vi "Read Temperature Controller Parameters.vi"(8 "error in (no error)":errorcluster, 11 "Temperature Controller Parameters in":refnum<class "Temperature Controller Parameters.lvclass">) -> (0 "error out":errorcluster, 2 "Data":T1={"Record heater"=FALSE, "Record RAW"=FALSE, "Set point"=0.0, "Heater range"=0.0, "Approach"=enum."Instant", "Ramp rate, K/min"=1.0, "Record Channels"=[], "Settling time "=60.0, "Settling range"=0.1, "P"=0.0, "I"=0.0, "D"=0.0, "Temperature Control"=FALSE}, 3 "Temperature Controller Parameters out":refnum<class "Temperature Controller Parameters.lvclass">)   [LabVIEW 2015, in "Temperature Controller Parameters.lvclass"]
uses:
  Temperature Controller Parameters.lvclass
  NHMFL_Core/Libraries/Instruments/Temperature Controller/Controls/T controller parameters.ctl
  NHMFL_Core/Libraries/Instruments/Temperature Controller/Controls/Set Point Aproach.ctl
panel:
  # "Temperature Monitor"
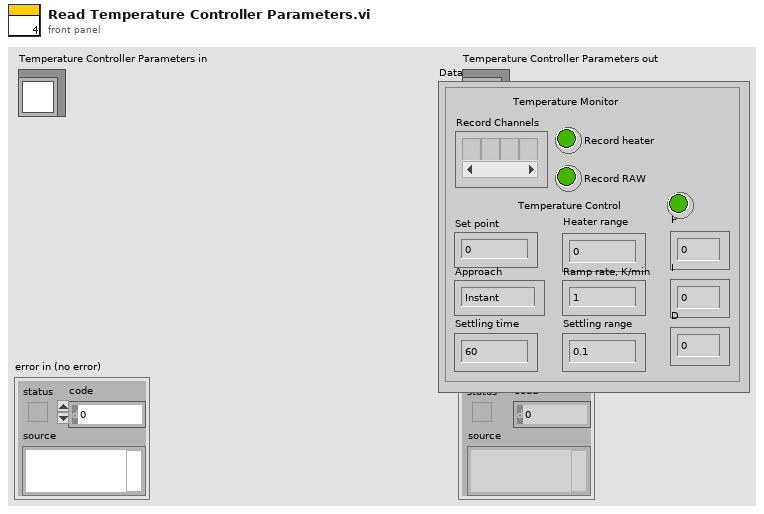
[diagram p1: front panel]
types:
  T1 = typedef "T controller parameters.ctl" = cluster{"Record heater":bool, "Record RAW":bool, "Set point":dbl, "Heater range":dbl, "Approach":T2, "Ramp rate, K/min":dbl, "Record Channels":string[], "Settling time ":dbl, "Settling range":dbl, "P":dbl, "I":dbl, "D":dbl, "Temperature Control":bool}
  T2 = typedef "Set Point Aproach.ctl" = enum16{"Instant", "Ramp"}
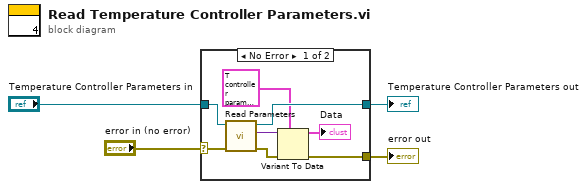
[diagram p0: block diagram]
diagram:
  n1 = case shown="No Error" "error in (no error)" {
    selector: "error in (no error)" -> [w10 w14]
    tunnel: [w5 w14] -> w3
    tunnel: [w11 w13] -> w1
    tunnel: "Temperature Controller Parameters in" -> [w12 w13]
    frame No Error {
      n2 = call-dynamic "Read Parameters.vi"("error in (no error)"=w10, "Mag Lab Parameters in"=w12) -> ("error out"=w6:errorcluster, "Parameters"=w9:variant, "Mag Lab Parameters out"=w11:refnum<class "Temperature Controller Parameters.lvclass">)  [unwired: 7 in]
      n3 = Variant To Data(error in=w6, type=T1 {"Record heater"=FALSE, "Record RAW"=FALSE, "Set point"=0.0, "Heater range"=0.0, "Approach"=enum."Instant", "Ramp rate, K/min"=0.0, "Record Channels"=[], "Settling time "=60.0, "Settling range"=0.1, "P"=0.0, "I"=0.0, "D"=0.0, "Temperature Control"=FALSE} ("Data"), Variant=w9) -> (data=→"Data":T1, error out=w5:errorcluster)
    }
    frame Error {
    }
  }
  "error out" <- w3
  "Temperature Controller Parameters out" <- w1
